vi "Close_Test.vi"(8 "error in (no error)":errorcluster caption="entrée d'erreur (pas d'erreur)", 11 "Test (Default) en entrée":refnum<class "Test (Default).lvclass">) -> (0 "error out":errorcluster caption="sortie d'erreur", 3 "Test (Default) en sortie":refnum<class "Test (Default).lvclass">)   [LabVIEW 2020, in "Library Test.lvlib" / "Test (Default).lvclass"]
uses:
  Test (Default).lvclass
  Test (Default).lvclass/Test (Default).ctl
  Core/Actors/Actor_Log/Actor_Log/Actor_Log Messages/Log Msg/Log Msg.lvclass/Log Msg.ctl
  <vilib>/ActorFramework/Message Enqueuer/Message Enqueuer.lvclass/Message Enqueuer.ctl
  <vilib>/ActorFramework/Message Enqueuer/Enqueue.vi
  Core/Actors/Actor_Log/Actor_Log/Actor_Log Messages/Log Msg/Log Msg.lvclass
  C:/Program Files (x86)/National Instruments/LabVIEW 2020/vi.lib/ActorFramework/Message/Message.lvclass
  <vilib>/ActorFramework/Message Priority Queue/Priority Enqueue.vi
  Commun VI/Library Commun.lvlib
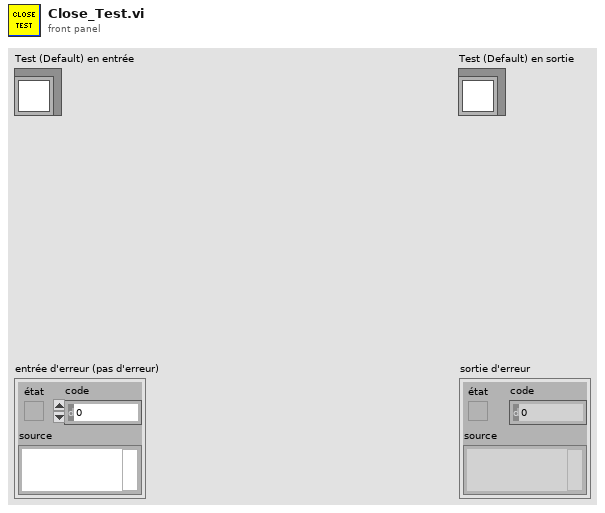
[diagram p1: front panel]
types:
  T1 = enum16{"Init", "Add Actor", "Delete Actor", "Get Actor Queue", "Get Log Actor Queue", "List all actors"}
  T2 = typedef "Library Commun.lvlib/Commande Type Test.ctl" = enum16{"Function", "Test", "Calculation"}
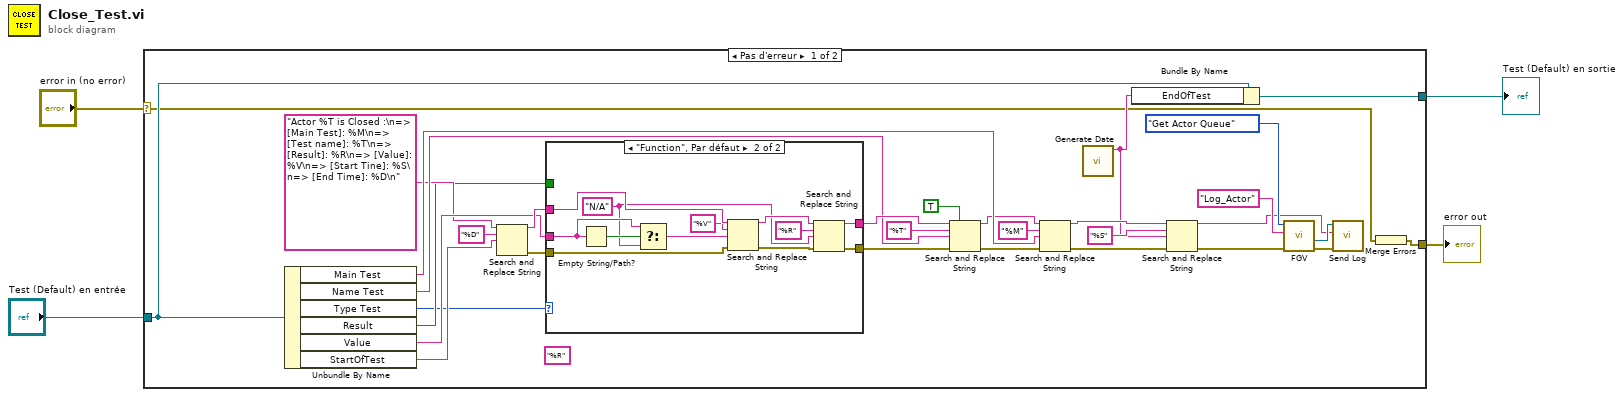
[diagram p0: block diagram]
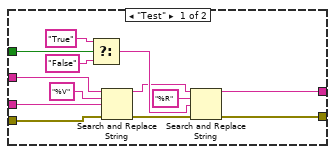
[diagram p2: hidden frame]
diagram:
  n1 = case shown="Pas d'erreur" "error in (no error)" {
    selector: "error in (no error)" -> [w9 w62]
    tunnel: [w8 w62] -> w2
    tunnel: [w35 w61] -> w3
    tunnel: "Test (Default) en entrée" -> [w21 w61]
    frame No Error {
      (unwired) "%R"
      n2 = Unbundle By Name(w21) -> ("Main Test"=w28:string, "Name Test"=w30:string, "Type Test"=w5:T2, "Result"=w6:bool, "Value"=w17:string, "StartOfTest"=w10:string)
      n3 = Search and Replace String(input string="Actor %T is Closed :\n=> [Main Test]: %M\n=> [Test name]: %T\n=> [Result]: %R\n=> [Value]: %V\n=> [Start Tine]: %S\n=> [End Time]: %D\n", search string="%D", replace string=w10) -> (result string=w20:string, error out=w19:errorcluster)  [unwired: 5 in, 2 out]
      n4 = case shown="\"Function\", Par défaut" w5 {
        tunnel: [w47 w60] -> w32
        tunnel: [w46 w59] -> w31
        tunnel: w20 -> [w42 w57]
        tunnel: w19 -> [w40 w55]
        tunnel: w17 -> [w37 w51]
        tunnel: w6 -> [w36 _]
        frame "Test" {
          n5 = Select(t="True", s=w36, f="False") -> (s? t:f=w48:string)
          n6 = Search and Replace String(input string=w42, search string="%V", replace string=w37, error in=w40) -> (result string=w41:string, error out=w39:errorcluster)  [unwired: 4 in, 2 out]
          n7 = Search and Replace String(input string=w41, search string="%R", replace string=w48, error in=w39) -> (result string=w46:string, error out=w47:errorcluster)  [unwired: 4 in, 2 out]
        }
        frame "Function", Default {
          w50 = "N/A"
          n8 = Empty String/Path?(string/path=w51) -> (empty?=w52:bool)
          n9 = Select(t=w51, s=w52, f=w50) -> (s? t:f=w49:string)
          n10 = Search and Replace String(input string=w57, search string="%V", replace string=w49, error in=w55) -> (result string=w56:string, error out=w54:errorcluster)  [unwired: 4 in, 2 out]
          n11 = Search and Replace String(input string=w56, search string="%R", replace string=w50, error in=w54) -> (result string=w59:string, error out=w60:errorcluster)  [unwired: 4 in, 2 out]
        }
      }
      n12 = Search and Replace String(replace all?=TRUE ("replace all? (F)"), input string=w31, search string="%T", replace string=w30, error in=w32) -> (result string=w27:string, error out=w29:errorcluster)  [unwired: 3 in, 2 out]
      n13 = Search and Replace String(input string=w27, search string="%M", replace string=w28, error in=w29) -> (result string=w14:string, error out=w16:errorcluster)  [unwired: 4 in, 2 out]
      n14 = call "Generate Date.vi"() -> ("chaîne de date/heure"=w11:string)  [unwired: 11 in]
      n15 = Bundle By Name(cluster=w21, "EndOfTest"=w11) -> (w35:refnum<class "Test (Default).lvclass">)
      n16 = Search and Replace String(input string=w14, search string="%S", replace string=w11, error in=w16) -> (result string=w13:string, error out=w15:errorcluster)  [unwired: 4 in, 2 out]
      n17 = call "FGV.vi"("error in (no error)"=w15, "Actor name"="Log_Actor", "Action"=T1."Get Actor Queue") -> ("error out"=w34:errorcluster, "Actor's Queue Out"=w33:refnum<class "Message Enqueuer.lvclass">)  [unwired: 6 in, 1 out]
      n18 = call "Send Log.vi"("error in (no error)"=w34, "String to add"=w13, "Message Enqueuer"=w33) -> ()  [unwired: 7 in, 2 out]
      n19 = Merge Errors(w9) -> (w8:errorcluster)
    }
    frame Error {
    }
  }
  "error out" <- w2
  "Test (Default) en sortie" <- w3
